vi "CMI ADS127L21 - Start Record.vi"(8 "error in (no error)":errorcluster, 11 "session in":T1 {"channels"."Channel" min=1 max=8 step=1; "channels"."Range [Vpk]" items=["±1.65V", "±2V"]}) -> (0 "error out":errorcluster, 3 "session out":T1 {"channels"."Channel" min=1 max=8 step=1; "channels"."Range [Vpk]" items=["±1.65V", "±2V"]})   [LabVIEW 2020]
doc: "Start recording."
uses:
  CMI ADS127L21 - Session.ctl
  CMI ADS127L21 - Record Channel.ctl
  CMI ADS127L21 - Input Range.ctl
  CMI ADS127L21 - Input Mode.ctl
  CMI ADS127L21 - Input Impedance.ctl
  CMI ADS127L21 - EXTOUT Mode.ctl
  CMI ADS127L21 - EXTOUT Polarity.ctl
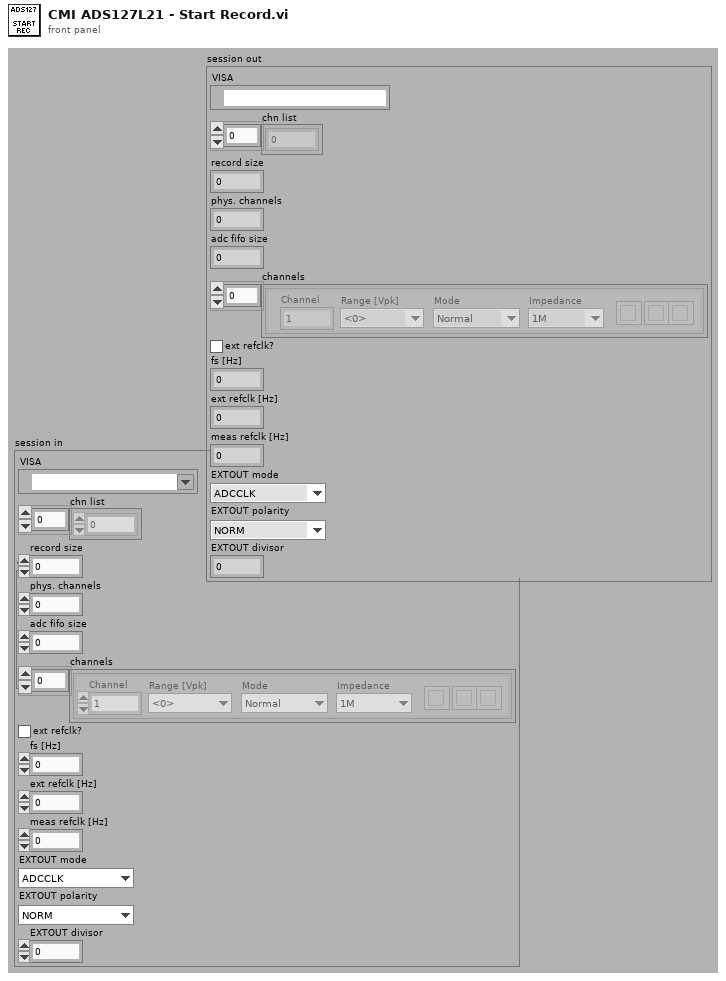
[diagram p1: front panel]
types:
  T1 = typedef "CMI ADS127L21 - Session.ctl" = cluster{"VISA":refnum<visa-resource-name>, "chn list":i32[], "record size":i32, "phys. channels":i32, "adc fifo size":i32, "channels":T2[], "ext refclk?":bool, "fs [Hz]":dbl, "ext refclk [Hz]":dbl, "meas refclk [Hz]":dbl, "EXTOUT mode":T6, "EXTOUT polarity":T7, "EXTOUT divisor":i32}
  T2 = typedef "CMI ADS127L21 - Record Channel.ctl" = cluster{"Range [Vpk]":T3, "Channel":i32, "Mode":T4, "Impedance":T5, "btn clr":bool, "btn up":bool, "btn down":bool}
  T3 = typedef "CMI ADS127L21 - Input Range.ctl" = dbl
  T4 = typedef "CMI ADS127L21 - Input Mode.ctl" = enum16{"Normal", "Inverted", "GND"}
  T5 = typedef "CMI ADS127L21 - Input Impedance.ctl" = enum16{"1M", "1k5"}
  T6 = typedef "CMI ADS127L21 - EXTOUT Mode.ctl" = enum16{"ADCCLK", "REFCLK", "SMPLCLK", "FIRST"}
  T7 = typedef "CMI ADS127L21 - EXTOUT Polarity.ctl" = enum16{"NORM", "INV"}
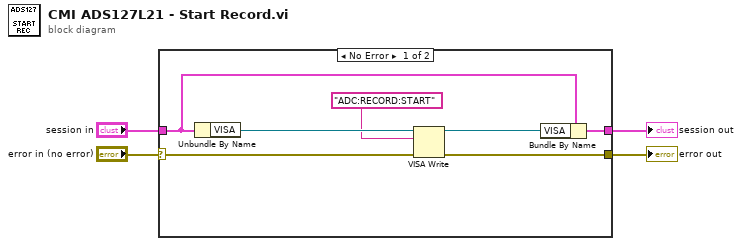
[diagram p0: block diagram]
diagram:
  n1 = case shown="No Error" "error in (no error)" {
    selector: "error in (no error)" -> [w5 w13]
    tunnel: "session in" -> [w9 w12]
    tunnel: [w10 w12] -> w3
    tunnel: [w8 w13] -> w2
    frame No Error {
      n2 = Unbundle By Name(w9) -> ("VISA"=w11:refnum<visa-resource-name>)
      n3 = VISA Write(VISA resource name=w11, write buffer="ADC:RECORD:START" ("format string"), error in (no error)=w5) -> (VISA resource name out=w7:refnum<visa-resource-name>, error out=w8:errorcluster)  [unwired: 1 out]
      n4 = Bundle By Name(cluster=w9, "VISA"=w7) -> (w10:T1)
    }
    frame Error {
    }
  }
  "error out" <- w2
  "session out" <- w3
